vi "Read Header Contents.vi"(8 "error in (no error)":errorcluster, 11 "Header in":refnum<class "Simulated_Header.lvclass">) -> (0 "error out":errorcluster, 2 "Header Content":T1, 3 "Header out":refnum<class "Simulated_Header.lvclass">)   [LabVIEW 2018, in "Simulated_Header.lvclass"]
uses:
  Simulated_Header.lvclass
  Simulated_Header.lvclass/Simulated_Header.ctl
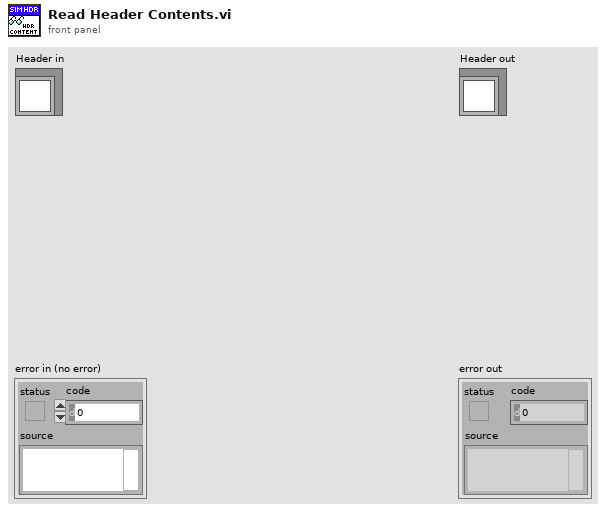
[diagram p1: front panel]
types:
  T1 = cluster{"FILENAME":cluster{"Name":string, "Value":string, "Comment":string}, "OBSERVER":cluster{"Name":string, "Value":string, "Comment":string}, "PROGRID":cluster{"Name":string, "Value":string, "Comment":string}, "OBJECT":cluster{"Name":string, "Value":string, "Comment":string}, "NIGHTDIR":cluster{"Name":string, "Value":string, "Comment":string}, "CHANNEL":cluster{"Name":string, "Value":string, "Comment":string}, "INSTRUME":cluster{"Name":string, "Value":string, "Comment":string}, "NEXPSEQ":cluster{"Name":string, "Value":string, "Comment":string}, "SEQINDEX":cluster{"Name":string, "Value":string, "Comment":string}, "OBSTYPE":cluster{"Name":string, "Value":string, "Comment":string}, "READMOD":cluster{"Name":string, "Value":string, "Comment":string}, "READMODE":cluster{"Name":string, "Value":string, "Comment":string}, "ACQMODE":cluster{"Name":string, "Value":string, "Comment":string}, "PREAMP":cluster{"Name":string, "Value":string, "Comment":string}, "READOUT":cluster{"Name":string, "Value":string, "Comment":string}, "VSHIFT":cluster{"Name":string, "Value":string, "Comment":string}, "TRIGGER":cluster{"Name":string, "Value":string, "Comment":string}, "EMMODE":cluster{"Name":string, "Value":string, "Comment":string}, "EMGAIN":cluster{"Name":string, "Value":string, "Comment":string}, "VBIN":cluster{"Name":string, "Value":string, "Comment":string}, "HBIN":cluster{"Name":string, "Value":string, "Comment":string}, "INITLIN":cluster{"Name":string, "Value":string, "Comment":string}, "INITCOL":cluster{"Name":string, "Value":string, "Comment":string}, "FINALLIN":cluster{"Name":string, "Value":string, "Comment":string}, "FINALCOL":cluster{"Name":string, "Value":string, "Comment":string}, "KSERLEN":cluster{"Name":string, "Value":string, "Comment":string}, "SHUTTER":cluster{"Name":string, "Value":string, "Comment":string}, "OPENSHT":cluster{"Name":string, "Value":string, "Comment":string}, "CLOSESHT":cluster{"Name":string, "Value":string, "Comment":string}, "DATE":cluster{"Name":string, "Value":string, "Comment":string}, "GAIN":cluster{"Name":string, "Value":string, "Comment":string}, "GAINERR":cluster{"Name":string, "Value":string, "Comment":string}, "RDNOISE":cluster{"Name":string, "Value":string, "Comment":string}, "RNOISERR":cluster{"Name":string, "Value":string, "Comment":string}, "SKYFIBER":cluster{"Name":string, "Value":string, "Comment":string}, "CALFIBER":cluster{"Name":string, "Value":string, "Comment":string}, "UTDATE":cluster{"Name":string, "Value":string, "Comment":string}, "LOCTIME":cluster{"Name":string, "Value":string, "Comment":string}, "MJD":cluster{"Name":string, "Value":string, "Comment":string}, "OBSLON":cluster{"Name":string, "Value":string, "Comment":string}, "OBSLAT":cluster{"Name":string, "Value":string, "Comment":string}, "OBSALT":cluster{"Name":string, "Value":string, "Comment":string}, "EXPTIME":cluster{"Name":string, "Value":string, "Comment":string}, "TELRA":cluster{"Name":string, "Value":string, "Comment":string}, "TELDEC":cluster{"Name":string, "Value":string, "Comment":string}, "RA":cluster{"Name":string, "Value":string, "Comment":string}, "DEC":cluster{"Name":string, "Value":string, "Comment":string}, "RA_DEG":cluster{"Name":string, "Value":string, "Comment":string}, "DEC_DEG":cluster{"Name":string, "Value":string, "Comment":string}, "EPOCH":cluster{"Name":string, "Value":string, "Comment":string}, "HA":cluster{"Name":string, "Value":string, "Comment":string}, "HAD":cluster{"Name":string, "Value":string, "Comment":string}, "AIRMASS":cluster{"Name":string, "Value":string, "Comment":string}, "AMSTART":cluster{"Name":string, "Value":string, "Comment":string}, "AMEND":cluster{"Name":string, "Value":string, "Comment":string}, "XOFFSET":cluster{"Name":string, "Value":string, "Comment":string}, "YOFFSET":cluster{"Name":string, "Value":string, "Comment":string}, "PA":cluster{"Name":string, "Value":string, "Comment":string}, "CAMFOC":cluster{"Name":string, "Value":string, "Comment":string}, "TELFOC":cluster{"Name":string, "Value":string, "Comment":string}, "TCSUT":cluster{"Name":string, "Value":string, "Comment":string}, "TCSST":cluster{"Name":string, "Value":string, "Comment":string}, "MOONDIST":cluster{"Name":string, "Value":string, "Comment":string}, "MOONALT":cluster{"Name":string, "Value":string, "Comment":string}, "MOONPHAS":cluster{"Name":string, "Value":string, "Comment":string}, "ADC":cluster{"Name":string, "Value":string, "Comment":string}, "ADCSPEED":cluster{"Name":string, "Value":string, "Comment":string}, "CALMIRR":cluster{"Name":string, "Value":string, "Comment":string}, "GUIDING":cluster{"Name":string, "Value":string, "Comment":string}, "GUIDTEXP":cluster{"Name":string, "Value":string, "Comment":string}, "GUIDFREQ":cluster{"Name":string, "Value":string, "Comment":string}, "GUIDOBJX":cluster{"Name":string, "Value":string, "Comment":string}, "GUIDOBJY":cluster{"Name":string, "Value":string, "Comment":string}, "AVGYCORR":cluster{"Name":string, "Value":string, "Comment":string}, "AVGXCORR":cluster{"Name":string, "Value":string, "Comment":string}, "GFOCUS":cluster{"Name":string, "Value":string, "Comment":string}, "THARLAMP":cluster{"Name":string, "Value":string, "Comment":string}, "HALLAMP":cluster{"Name":string, "Value":string, "Comment":string}, "AGITATOR":cluster{"Name":string, "Value":string, "Comment":string}, "THARMIRR":cluster{"Name":string, "Value":string, "Comment":string}, "DSTATUS":cluster{"Name":string, "Value":string, "Comment":string}, "DPOS":cluster{"Name":string, "Value":string, "Comment":string}, "DTEMP":cluster{"Name":string, "Value":string, "Comment":string}, "DHUM":cluster{"Name":string, "Value":string, "Comment":string}, "DLAMP":cluster{"Name":string, "Value":string, "Comment":string}, "DFLAT":cluster{"Name":string, "Value":string, "Comment":string}, "TEMPEXT":cluster{"Name":string, "Value":string, "Comment":string}, "PRESSURE":cluster{"Name":string, "Value":string, "Comment":string}, "HUMIDITY":cluster{"Name":string, "Value":string, "Comment":string}, "WINDDIR":cluster{"Name":string, "Value":string, "Comment":string}, "WINSPEED":cluster{"Name":string, "Value":string, "Comment":string}, "SHTTTL":cluster{"Name":string, "Value":string, "Comment":string}, "COOLER":cluster{"Name":string, "Value":string, "Comment":string}, "TEMP":cluster{"Name":string, "Value":string, "Comment":string}, "TEMPST":cluster{"Name":string, "Value":string, "Comment":string}, "SERN":cluster{"Name":string, "Value":string, "Comment":string}, "OBS_TITLE":cluster{"Name":string, "Value":string, "Comment":string}, "COMMENT":cluster{"Name":string, "Value":string, "Comment":string}}
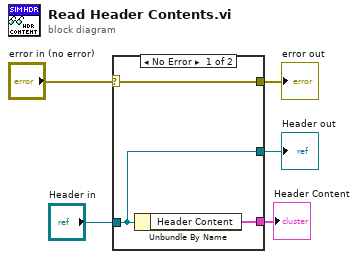
[diagram p0: block diagram]
diagram:
  n1 = case shown="No Error" "error in (no error)" {
    selector: "error in (no error)" -> [w8 w9]
    tunnel: [w8 w9] -> w4
    tunnel: [w7 w10] -> w2
    tunnel: "Header in" -> [w7 w10]
    tunnel: [w6 _] -> w1
    frame No Error {
      n2 = Unbundle By Name(w7) -> ("Header Content"=w6:T1)
    }
    frame Error {
    }
  }
  "error out" <- w4
  "Header out" <- w2
  "Header Content" <- w1
